vi "Home.vi"(8 "error in (no error)":errorcluster, 9 "mode":i32, 10 "axisNumber":i32, 11 "reference":refnum<k24>) -> (0 "error out":errorcluster, 3 ".NET Refnum out":refnum<k24>)   [LabVIEW 2019, in "ESP301-Driver.lvlib"]
uses:
  ESP301-Driver.lvlib
  Newport.ESP301.CommandInterface
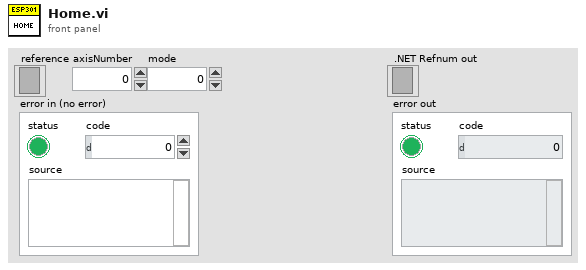
[diagram p1: front panel]
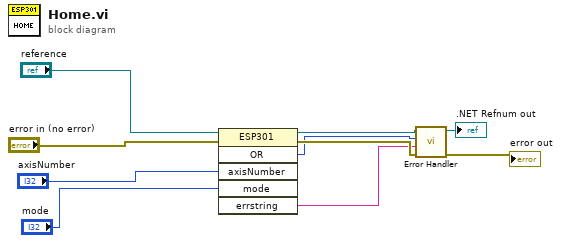
[diagram p0: block diagram]
diagram:
  n1 = invoke class="ESP301" method="OR"(reference="reference", error in="error in (no error)", "axisNumber"="axisNumber", "mode"="mode") -> (reference out=w6:refnum<k24>, error out=w5:errorcluster, "OR"=w4:i32, "errstring"=w3:string)  [unwired: 2 in, 2 out]
  n2 = call "Error Handler.vi"("error in (no error)"=w5, "Message"=w3, "Error Code"=w4, ".NET Refnum in"=w6) -> ("error out"=→"error out":errorcluster, ".NET Refnum out"=→".NET Refnum out":refnum<k24>)  [unwired: 6 in]
